vi "Update Advanced Timing Visibility.vi"(10 "Previous UI Data in":refnum<class "Settings UI.lvclass">, 11 "New UI Data in":refnum<class "Settings UI.lvclass">) -> (2 "Previous UI Data out":refnum<class "Settings UI.lvclass">, 3 "New UI Data out":refnum<class "Settings UI.lvclass">)   [LabVIEW 2024, in "Output Sequencer.lvlib" / "Settings UI.lvclass"]
uses:
  Settings UI.lvclass
  Types/Tree Index Enum.ctl
  Settings UI.lvclass/Settings UI.ctl
  Globals/Global Tree Data.vi
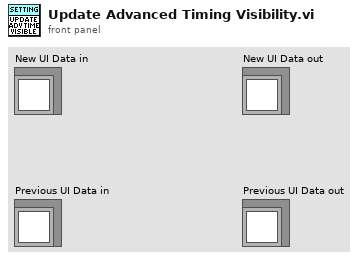
[diagram p1: front panel]
types:
  T1 = typedef "Output Sequencer.lvlib/Settings UI.lvclass/Tree Index Enum.ctl" = enum16{"General Settings", "Num Steps", "Num Analog", "Num Digital", "Show Confirmation", "Interp Priority", "Adv Timing", "Enable Conditions", "Seq Execution", "Reset Test Start", "Only When Test", "Delay After Test", "Start condition", "Re-triggering", "Stop condition", "Stop After Cycles", "Stop Values", "Default Values", "Default Analog", "Default Digital", "Steps", "Step #", "Description", "Precondition", "Duration", "Mode", "Delay Between Vals", "Analog Values", "Digital Values", "Postcondition", "On True", "On False"}
  T2 = typedef "Output Sequencer.lvlib/Settings UI.lvclass/Step Settings.ctl" = cluster{"Description":string, "Precondition":string, "Duration":dbl, "Mode":string, "Delay Between Values":dbl, "Analog Values":string[], "Digital Values":string[], "Postcondition":string, "On True":string, "On False":string}
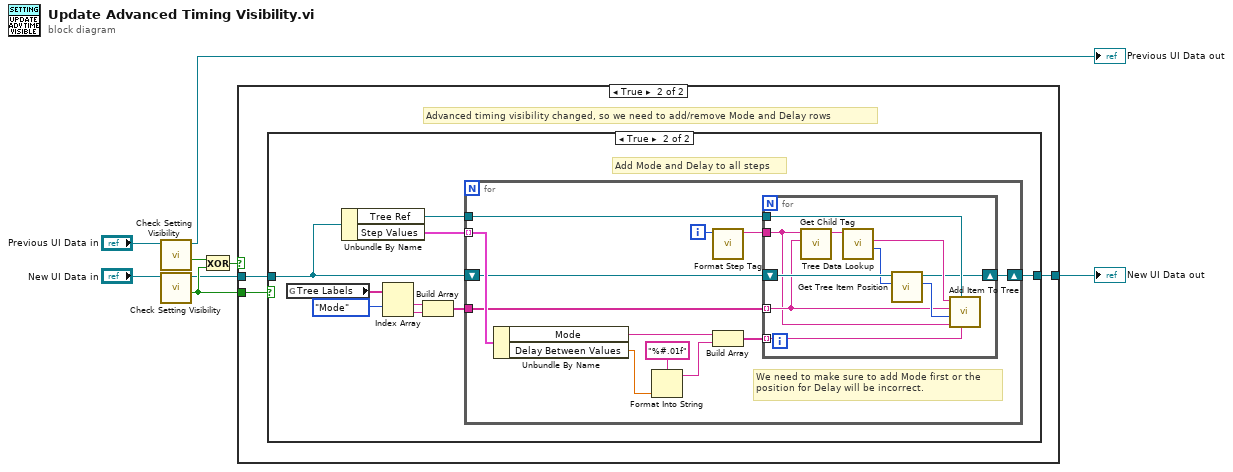
[diagram p0: block diagram]
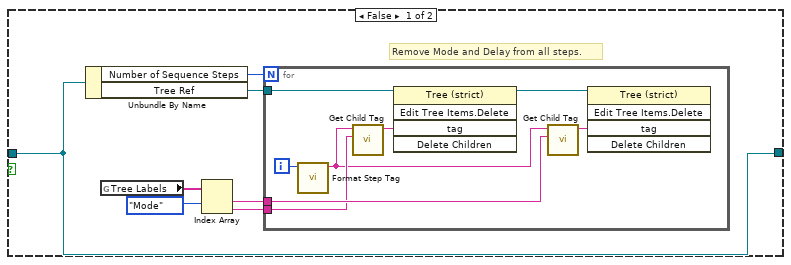
[diagram p3: hidden frame]
diagram:
  n1 = call "Check Setting Visibility.vi"("UI Data in"="Previous UI Data in") -> ("Advanced timing visible"=w6:bool, "UI Data out"=→"Previous UI Data out":refnum<class "Settings UI.lvclass">)  [unwired: 7 in, 2 out]
  n2 = call "Check Setting Visibility.vi"("UI Data in"="New UI Data in") -> ("Advanced timing visible"=w5:bool, "UI Data out"=w4:refnum<class "Settings UI.lvclass">)  [unwired: 7 in, 2 out]
  n3 = Exclusive Or(1:w5, 2:w6) -> (0:w8:bool)
  n4 = case shown="True" w8 {
    tunnel: w5 -> [_ w12]
    tunnel: w4 -> [w9 w11]
    tunnel: [w9 w10] -> w3
    frame False {
      # "Change didn't affect if we should or should not display Mode and Delay"
    }
    frame True {
      # "Advanced timing visibility changed, so we need to add/remove Mode and Delay rows"
      n5 = case shown="True" w12 {
        tunnel: w11 -> [w13 w34]
        tunnel: [w13 w29] -> w10
        frame False {
          # "Remove Mode and Delay from all steps."
          n6 = Unbundle By Name(w13) -> ("Number of Sequence Steps"=w14:i32, "Tree Ref"=w15:refnum<vi>)
          n7 = global read "Global Tree Data.vi" "Tree Labels"() -> (w19:string[])
          n8 = Index Array(array=w19, index #1=Tree_Index_Enum."Mode" ("Tree Index Enum")) -> (element #1=w17:string, element #2=w16:string)  [unwired: 1 in]
          n9 = for {
            N: w14 -> [_]
            tunnel: w17 -> [w24]
            tunnel: w16 -> [w23]
            tunnel: w15 -> [w20]
            i -> [w22]
            n10 = call "Format Step Tag.vi"("Step Number"=w22) -> ("Tag"=w21:string)  [unwired: 10 in]
            n11 = call "Get Child Tag.vi"("Child label"=w23, "Parent tag"=w21) -> ("Child tag"=w25:string)  [unwired: 9 in]
            n12 = invoke class="Tree (strict)" method="Edit Tree Items.Delete"(reference=w20, "tag"=w25) -> (reference out=w27:refnum<vi>)  [unwired: 3 in, 4 out]
            n13 = call "Get Child Tag.vi"("Child label"=w24, "Parent tag"=w21) -> ("Child tag"=w26:string)  [unwired: 9 in]
            n14 = invoke class="Tree (strict)" method="Edit Tree Items.Delete"(reference=w27, "tag"=w26) -> ()  [unwired: 3 in, 5 out]
          }
        }
        frame True {
          # "Add Mode and Delay to all steps"
          n15 = global read "Global Tree Data.vi" "Tree Labels"() -> (w36:string[])
          n16 = Unbundle By Name(w34) -> ("Tree Ref"=w28:refnum<vi>, "Step Values"=w33:T2[])
          n17 = Index Array(array=w36, index #1=Tree_Index_Enum."Mode" ("Tree Index Enum")) -> (element #1=w32:string, element #2=w31:string)  [unwired: 1 in]
          n18 = Build Array(w32, w31) -> (w30:string[])
          n19 = for {
            tunnel: w33 -> [w48] mode=indexing
            tunnel: w28 -> [w43]
            tunnel: w30 -> [w38]
            shift-right: [w37] -> w29
            shift-left: w34 -> [w41]
            i -> [w40]
            # "We need to make sure to add Mode first or the\nposition for Delay will be incorrect."
            n20 = Unbundle By Name(w48) -> ("Mode"=w44:string, "Delay Between Values"=w47:dbl)
            n21 = Format Into String(format string="%#.01f", w47) -> (resulting string=w45:string)  [unwired: 2 in, 1 out]
            n22 = call "Format Step Tag.vi"("Step Number"=w40) -> ("Tag"=w39:string)  [unwired: 10 in]
            n23 = Build Array(w44, w45) -> (w42:string[])
            n24 = for {
              tunnel: w39 -> [w53]
              tunnel: w38 -> [w55] mode=indexing
              tunnel: w43 -> [w54]
              tunnel: w42 -> [w52] mode=indexing
              shift-right: [w49] -> w37
              shift-left: w41 -> [w58]
              n25 = call "Get Child Tag.vi"("Child label"=w55, "Parent tag"=w53) -> ("Child tag"=w51:string)  [unwired: 9 in]
              n26 = call "Tree Data Lookup.vi"("Tag in"=w51) -> ("Tree Index Enum"=w57:T1, "Tag out"=w50:string)  [unwired: 5 in, 4 out]
              n27 = call "Get Tree Item Position.vi"("Step item"=w57, "UI Data in"=w58) -> ("Position"=w56:i32, "UI Data out"=w49:refnum<class "Settings UI.lvclass">)  [unwired: 8 in]
              n28 = call "Add Item To Tree.vi"("Child Text"=w52, "TreeControl in"=w54, "Parent Tag"=w53, "Child Position"=w56, "Left Cell String"=w55, "Child Tag in"=w50) -> ()  [unwired: 5 in, 1 out]
            }
          }
        }
      }
    }
  }
  "New UI Data out" <- w3
